vi "meteo.vi"(0 "ComPort 2":i16=3) -> (1 "Wind Speed 2":i16(knob) scale=0.0..25.0, 2 "Wind Angle 2":sgl(knob) scale=0.0..360.0, 3 "Direction 2":string, 4 "Outside Temperature":sgl, 5 "Inside Temp":sgl, 6 "Solar":i16, 7 "UV":sgl)   [LabVIEW 2012]
uses:
  libs/VantagePro/VantagePro.lvlib
panel:
  out "error out 2":errorcluster
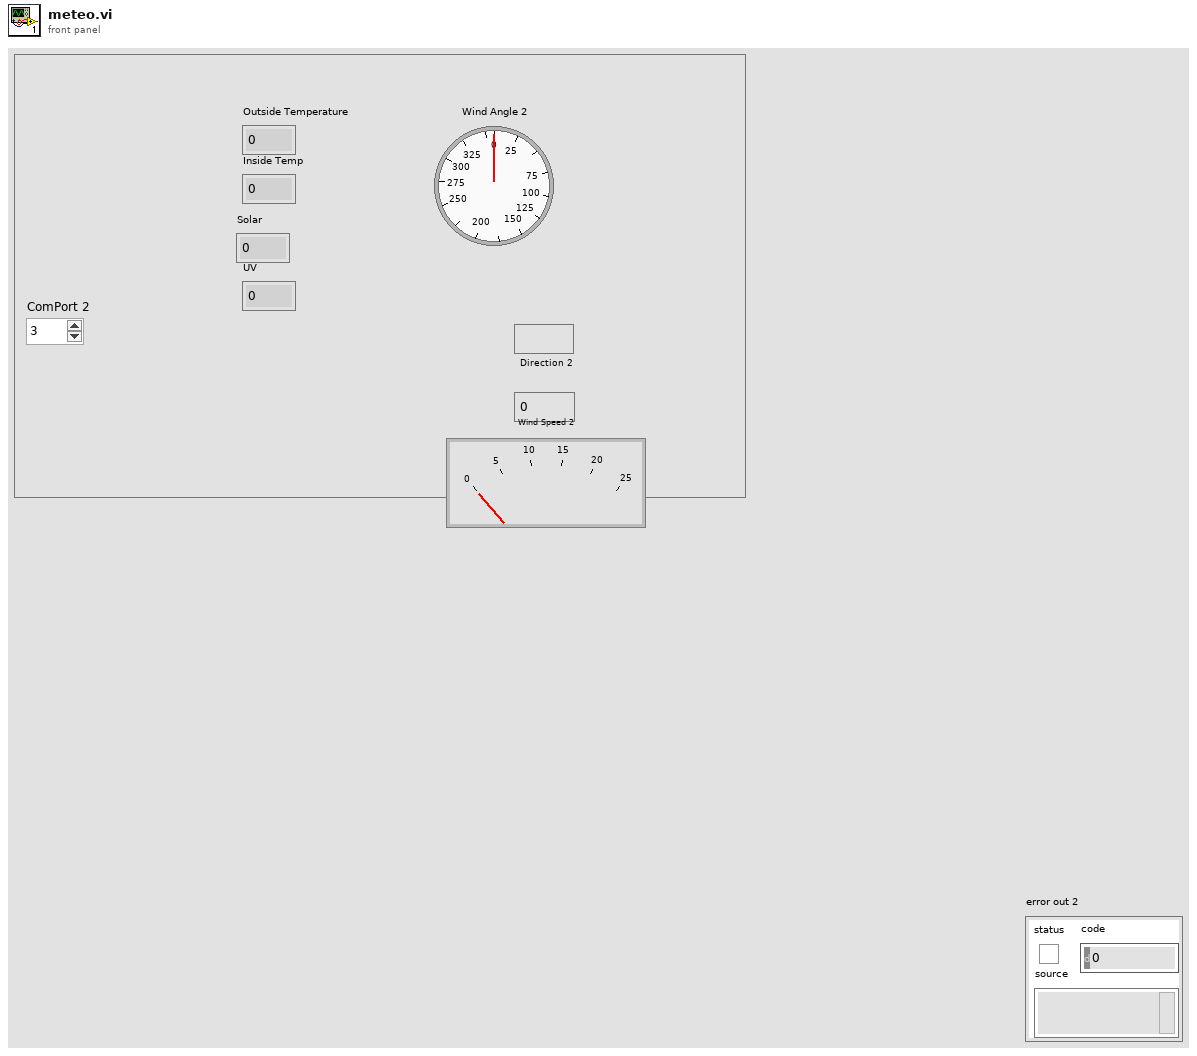
[diagram p1: front panel]
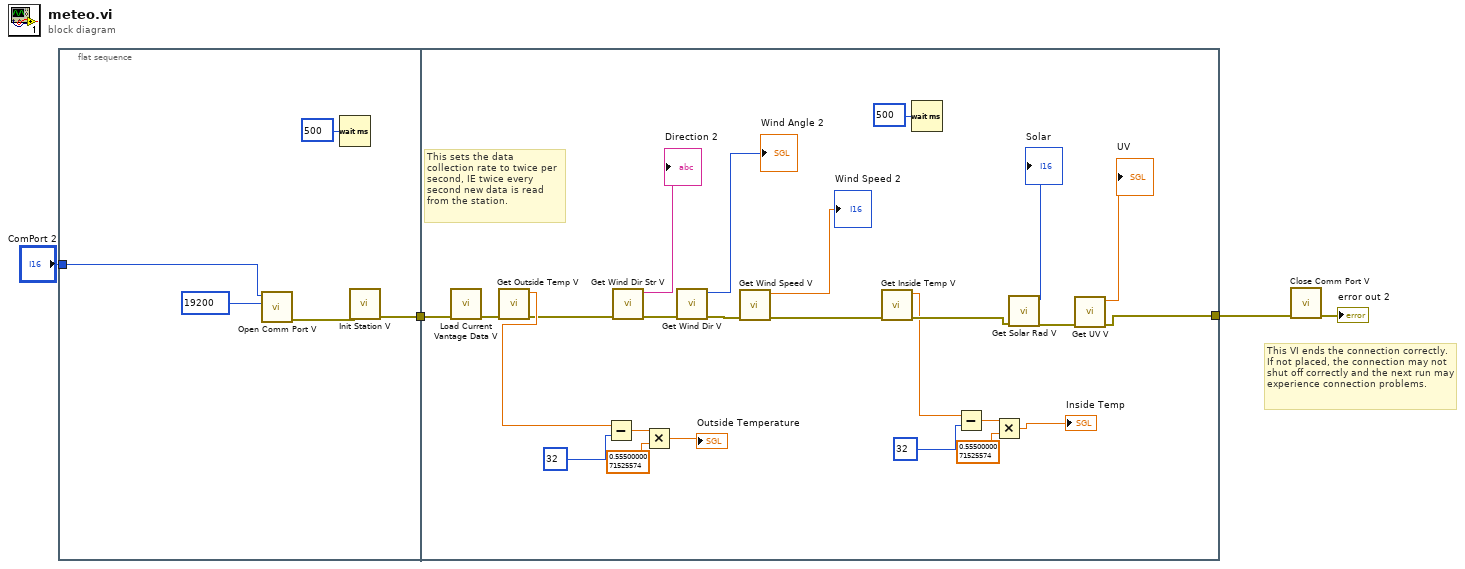
[diagram p0: block diagram]
diagram:
  # "This VI ends the connection correctly. If not placed, the connection may not shut off correctly and the next run may experience connection problems."
  n1 = flat-sequence {
    tunnel: "ComPort 2" -> [w7]
    tunnel: [w6] -> w3
    tunnel: w3 -> [w28]
    tunnel: [w22] -> w2
    frame #0 {
      n2 = call "Open Comm Port V.vi"("baudRate"=19200, "comPort"=w7) -> ("error out"=w8:errorcluster)  [unwired: 8 in, 1 out]
      n3 = Wait (ms)(milliseconds to wait=u32 500) -> ()  [unwired: 1 out]
      n4 = call "Init Station V.vi"("error in (no error)"=w8) -> ("error out"=w6:errorcluster)  [unwired: 9 in, 1 out]
    }
    frame #1 {
      # "This sets the data collection rate to twice per second, IE twice every second new data is read from the station."
      n5 = call "Load Current Vantage Data V.vi"("error in (no error)"=w28) -> ("error out"=w34:errorcluster)  [unwired: 9 in, 1 out]
      n6 = call "Get Outside Temp V.vi"("error in (no error)"=w34) -> ("error out"=w10:errorcluster, "function return"=w18:sgl)  [unwired: 9 in]
      n7 = Subtract(x=w18, y=32) -> (x-y=w20:sgl)
      n8 = call "Get Wind Dir Str V.vi"("error in (no error)"=w10) -> ("error out"=w31:errorcluster, "dirStr out"=→"Direction 2":string)  [unwired: 8 in, 1 out]
      n9 = Multiply(x=w20, y=sgl 0.555) -> (x*y=→"Outside Temperature":sgl)
      n10 = call "Get Wind Dir V.vi"("error in (no error)"=w31) -> ("error out"=w30:errorcluster, "function return"=→"Wind Angle 2":i16)  [unwired: 9 in]
      n11 = call "Get Wind Speed V.vi"("error in (no error)"=w30) -> ("error out"=w27:errorcluster, "function return"=→"Wind Speed 2":sgl)  [unwired: 9 in]
      n12 = call "Get Inside Temp V.vi"("error in (no error)"=w27) -> ("error out"=w26:errorcluster, "function return"=w13:sgl)  [unwired: 9 in]
      n13 = Wait (ms)(milliseconds to wait=u32 500) -> ()  [unwired: 1 out]
      n14 = Subtract(x=w13, y=32) -> (x-y=w15:sgl)
      n15 = Multiply(x=w15, y=sgl 0.555) -> (x*y=→"Inside Temp":sgl)
      n16 = call "Get Solar Rad V.vi"("error in (no error)"=w26) -> ("error out"=w24:errorcluster, "function return"=→"Solar":i16)  [unwired: 9 in]
      n17 = call "Get UV V.vi"("error in (no error)"=w24) -> ("error out"=w22:errorcluster, "function return"=→"UV":sgl)  [unwired: 9 in]
    }
  }
  n18 = call "Close Comm Port V.vi"("error in (no error)"=w2) -> ("error out"=→"error out 2":errorcluster)  [unwired: 9 in, 1 out]
